vi "Do.vi"(8 "error in (no error)":errorcluster, 10 "Actor in":refnum<class "Actor.lvclass">, 11 "Replay Message":refnum<class "Replay Msg.lvclass">) -> (0 "error out":errorcluster, 2 "Actor out":refnum<class "Actor.lvclass">)   [LabVIEW 2014, in "Replay Msg.lvclass"]
doc: "(<B>Filename</B>: Actor Framework.lvlib:Message.lvclass:Do.vi)\n\nDefines what a message does when it is received by an actor. Generally, a message instructs an actor to invoke one of its methods. By default, this method does nothing. A child class must override it to define behavior. Create a child class by using the Actor Framework Message Maker dialog box."
uses:
  Replay Msg.lvclass
  <vilib>/ActorFramework/Actor/Actor.lvclass
  Replay Msg.lvclass/Replay Msg.ctl
  <vilib>/ActorFramework/Message Enqueuer/Message Enqueuer.lvclass/Message Enqueuer.ctl
  <vilib>/ActorFramework/Message Priority Queue/Priority Enqueue.vi
  <vilib>/ActorFramework/Message Enqueuer/Message Enqueuer.lvclass
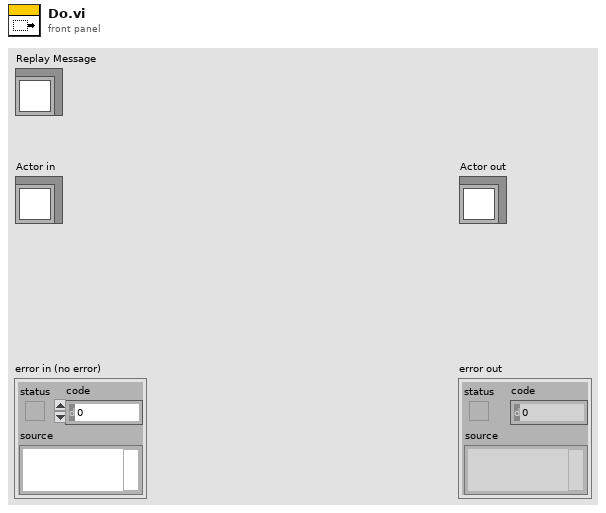
[diagram p1: front panel]
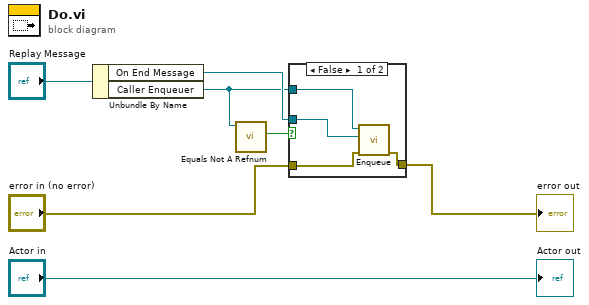
[diagram p0: block diagram]
diagram:
  n1 = Unbundle By Name("Replay Message") -> ("On End Message"=w5:refnum<class "Message.lvclass">, "Caller Enqueuer"=w4:refnum<class "Message Enqueuer.lvclass">)
  n2 = call <vilib>:"Equals Not A Refnum.vi"("Message Enqueuer"=w4) -> ("Not a refnum?"=w6:bool)  [unwired: 10 in]
  n3 = case shown="False" w6 {
    tunnel: w5 -> [w11 _]
    tunnel: w4 -> [w10 _]
    tunnel: "error in (no error)" -> [w9 w12]
    tunnel: [w8 w12] -> w2
    frame False {
      n4 = call <vilib>:"Enqueue.vi"("error in (no error)"=w9, "Message"=w11, "Message Enqueuer in"=w10) -> ("error out"=w8:errorcluster)  [unwired: 7 in, 1 out]
    }
    frame True {
    }
  }
  "error out" <- w2
  "Actor out" <- "Actor in"
